vi "Write Name.vi"(8 "error in (no error)":errorcluster, 10 "Name":string, 11 "Message Transport Interface in":refnum<class "Message Transport Interface.lvclass">) -> (0 "error out":errorcluster, 3 "Message Transport Interface out":refnum<class "Message Transport Interface.lvclass">)   [LabVIEW 2016, in "Stream Mediator.lvlib" / "Message Transport Interface.lvclass"]
doc: "--\nCopyright © 2017 Composed SystemsI All rights reserved.\n\nAuthor: Jon McBee <jon.mcbee@composed.io>\n\nThis library is provided \"AS IS\" ,WITHOUT WARRANTIES OR\nCONDITIONS OF ANY KIND, either express or implied.\n\nComposed Systems -- composed.io\n\nStream 0.0.1.1\nJon McBee - Composed Systems\nCopyright (c) 2017, Composed Systems"
uses:
  <userlib>/Composed Systems/Stream/Mediator/Classes/Message Transport Interface/Message Transport Interface.lvclass
  <userlib>/Composed Systems/Stream/Mediator/Classes/Message Transport Interface/Message Transport Interface.lvclass/Message Transport Interface.ctl
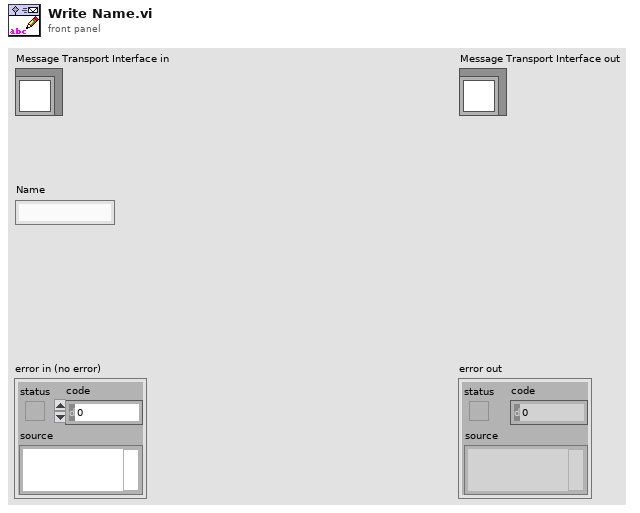
[diagram p1: front panel]
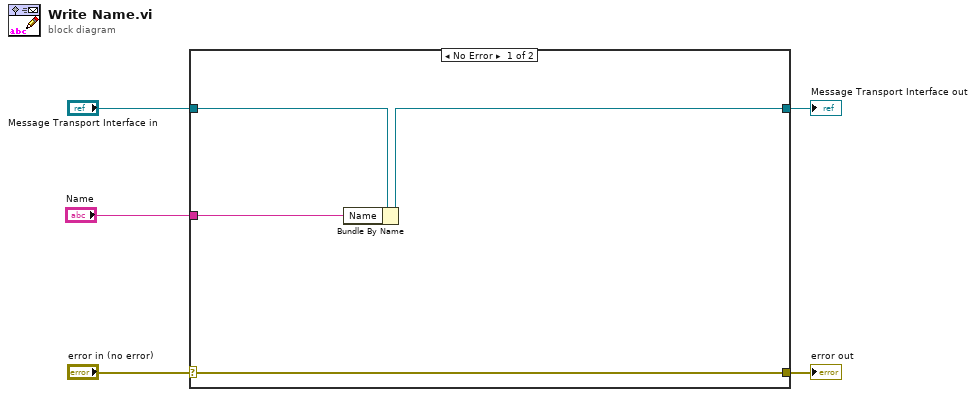
[diagram p0: block diagram]
diagram:
  n1 = case shown="No Error" "error in (no error)" {
    selector: "error in (no error)" -> [w9 w11]
    tunnel: [w9 w11] -> w4
    tunnel: [w6 w10] -> w2
    tunnel: "Message Transport Interface in" -> [w7 w10]
    tunnel: "Name" -> [w8 _]
    frame No Error {
      n2 = Bundle By Name(cluster=w7, "Name"=w8) -> (w6:refnum<class "Message Transport Interface.lvclass">)
    }
    frame Error {
    }
  }
  "error out" <- w4
  "Message Transport Interface out" <- w2
